vi "Write Graph Data.vi"(10 "Graph Data":cluster{"Array":dbl[], "Array":dbl[]}[](array[cluster]), 11 "AM-AM in":refnum<class "AM-AM.lvclass">) -> (3 "AM-AM out":refnum<class "AM-AM.lvclass">)   [LabVIEW 2020, in "AM-AM.lvclass"]
uses:
  AM-AM.lvclass
  AM-AM.lvclass/AM-AM.ctl
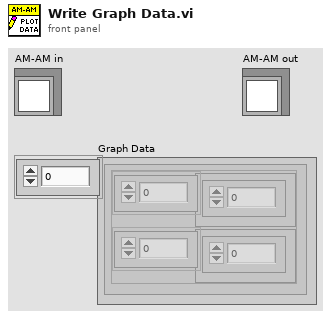
[diagram p1: front panel]
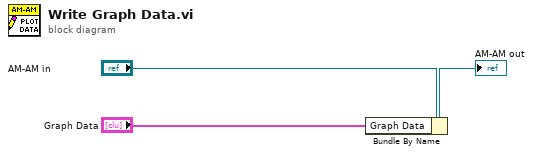
[diagram p0: block diagram]
diagram:
  n1 = Bundle By Name(cluster="AM-AM in", "Graph Data"="Graph Data") -> (→"AM-AM out":refnum<class "AM-AM.lvclass">)
